vi "ParsingFitFormulae.vi"(1 "String":string="\nf%d(t) = cmax%d*((t/xmax%d)**(-(1+m%d)*q%d)*exp(((1+m%d)/2)*(1-(t/xmax%d)**(-2*q%d))))\ncmax%d = %.2f; xmax%d = %.2f; m%d = 1;  q%d = 0.73         # initial guess for cmax and xmax q and m\nfit f%d(t) \"%s.dat\" index %d using %s via cmax%d, xmax%d, m%d, q%d  #this is a gaussian fit\n") -> (0 "element":string)   [LabVIEW 2022 SP3]
uses:
  <vilib>/regexp/Match Regular Expression.xnode
panel:
  out "Numeric":i32
  out "Array":string[](array[string])
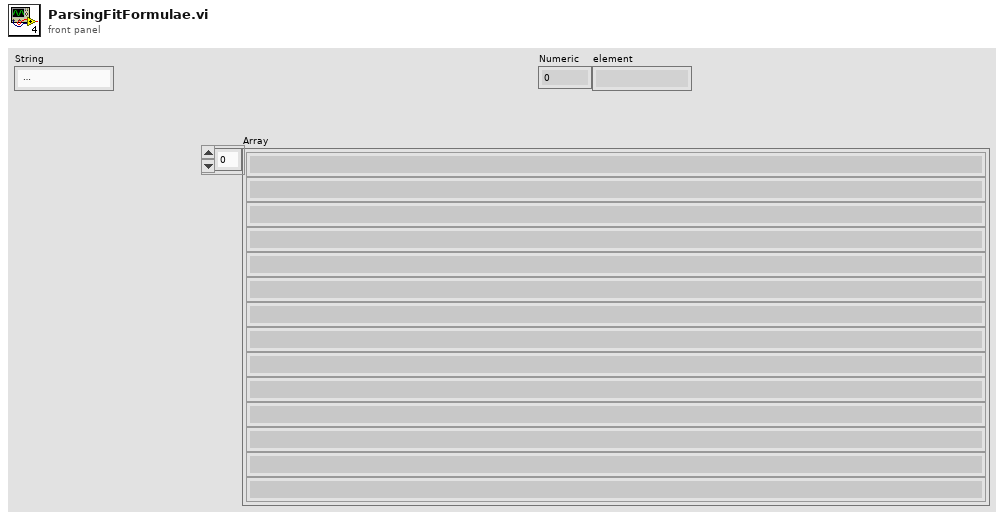
[diagram p1: front panel]
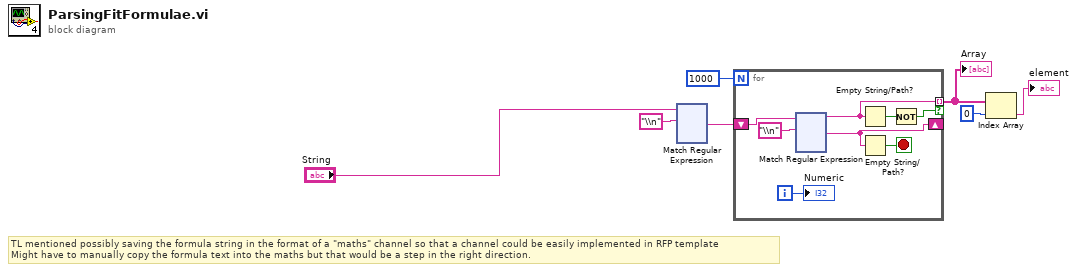
[diagram p0: block diagram]
diagram:
  # "TL mentioned possibly saving the formula string in the format of a \"maths\" channel so that a channel could be easily implemented in RFP template\nMight have to manually copy the formula text into the maths but that would be a step in the right direction."
  n1 = xnode "Match Regular Expression"("input string"="String", "regular expression"="\\n") -> ("after match"=w4:string)  [unwired: 4 in, 4 out]
  n2 = for {
    N: 1000 -> [_]
    shift-right: [w9] -> _
    shift-left: w4 -> [w15]
    tunnel: [w13] -> w3 mode=indexing if=w12
    i -> [w10]
    stop <- w8 stop-if-true
    # "Scan more than enough lines to get all of the Registers' string descriptions arranged into an array"
    n3 = xnode "Match Regular Expression"("input string"=w15, "regular expression"="\\n") -> ("before match"=w13:string, "after match"=w9:string)  [unwired: 4 in, 3 out]
    n4 = Empty String/Path?(string/path=w13) -> (empty?=w11:bool)
    n5 = Empty String/Path?(string/path=w9) -> (empty?=w8:bool)
    n6 = Not(x=w11) -> (.not. x?=w12:bool)
    "Numeric" <- w10
  }
  "Array" <- w3
  n7 = Index Array(array=w3, index=0) -> (element=→"element":string)
